vi "NI-Switch Main Page.vi"(8 "error in (no error)":errorcluster, 11 "Node Ptr":T1 format="%.0x") -> (0 "error out":errorcluster)   [LabVIEW 2010, in "NI-Switch Relay Custom Device.lvlib"]
uses:
  NI-Switch Relay Custom Device.lvlib
  <vilib>/NI Veristand/Custom Device API/Custom Device Item Ref.ctl
  NI-Switch Global.vi
  <vilib>/NI Veristand/Custom Device API/Get Item Property (String).vi
  <vilib>/NI Veristand/Custom Device API/Set Item Property (String).vi
  <vilib>/NI Veristand/Custom Device API/Custom Device API.lvlib
panel:
  out "Topology Name":string
  in  "Header 3":cluster{"Section Name":string}={"Section Name"="Custom Device Item Settings"}
  in  "Physical Address":string
  in  "Decimation":i32
  in  "Header 2":cluster{"Section Name":string}={"Section Name"="Custom Device Item Settings"}
  in  "Header":cluster{"Section Name":string}={"Section Name"="Custom Device Item Settings"}
  in  "Description":string
  in  "Name":string
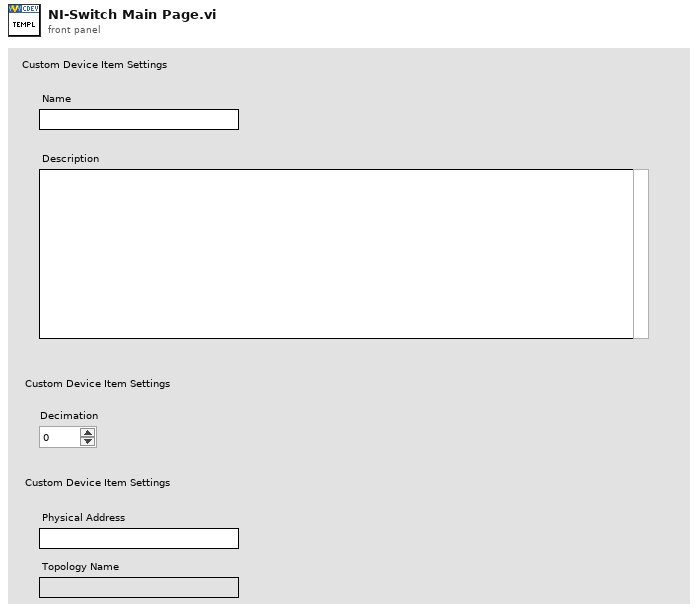
[diagram p1: front panel]
types:
  T1 = typedef "Custom Device API.lvlib/Custom Device Item Ref.ctl" = u64
  T2 = typedef "Custom Device API.lvlib/Custom Device Item Info.ctl" = cluster{"Name":string, "Is Channel":bool, "GUID":string}
  T3 = typedef "Custom Device API.lvlib/Custom Device Commands.ctl" = enum16{"Default", "Item renamed", "Shutdown", "Dynamic button pressed"}
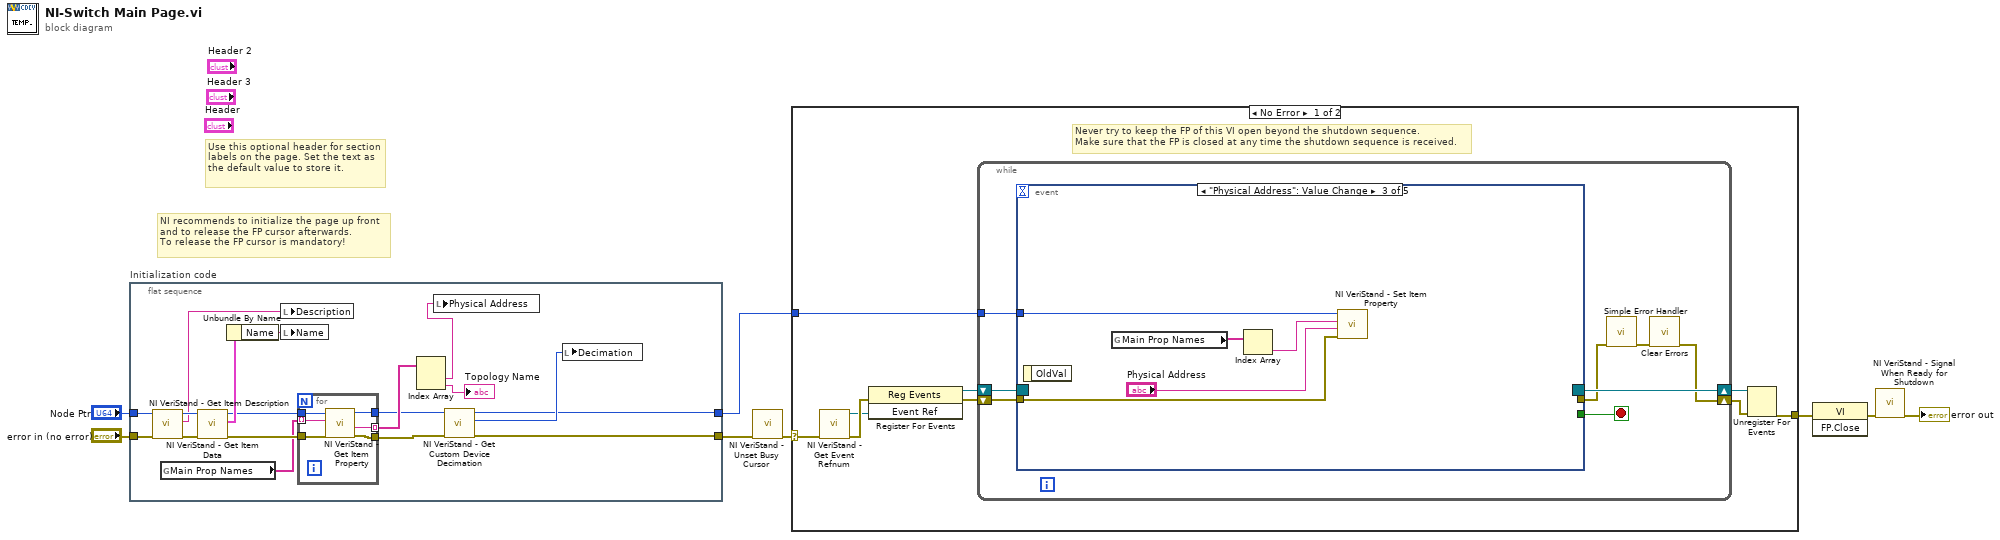
[diagram p0: block diagram]
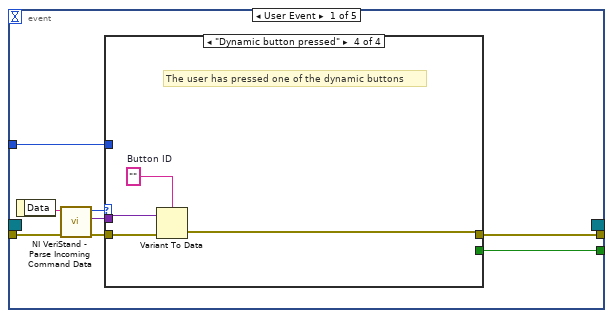
[diagram p2: hidden frame]
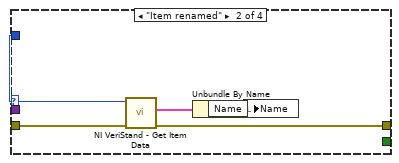
[diagram p4: hidden frame]
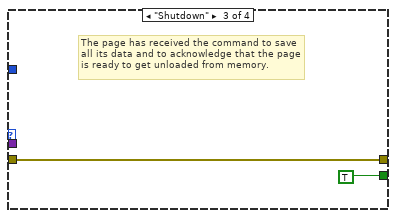
[diagram p5: hidden frame]
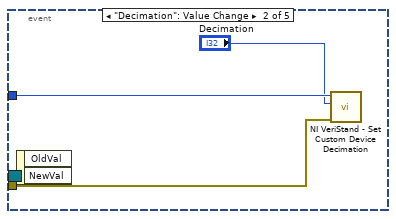
[diagram p6: hidden frame]
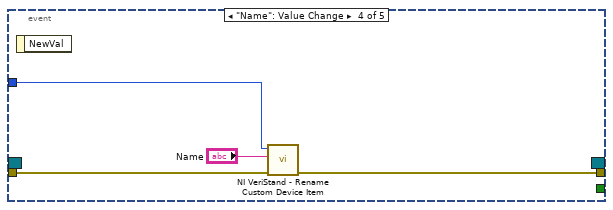
[diagram p7: hidden frame]
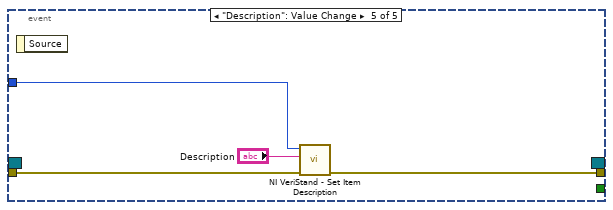
[diagram p8: hidden frame]
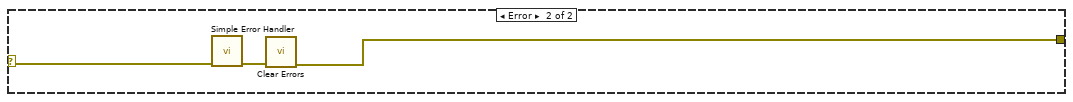
[diagram p9: hidden frame]
diagram:
  # "Use this optional header for section labels on the page. Set the text as the default value to store it."
  # "NI recommends to initialize the page up front\nand to release the FP cursor afterwards.\nTo release the FP cursor is mandatory!"
  n1 = flat-sequence "Initialization code" {
    tunnel: "error in (no error)" -> [w25]
    tunnel: "Node Ptr" -> [w24]
    tunnel: [w9] -> w4
    tunnel: [w10] -> w1
    frame #0 {
      n2 = call <vilib>:"NI VeriStand - Get Item Description.vi"("error in (no error)"=w25, "Item Ref in"=w24) -> ("error out"=w22:errorcluster, "Description"=w23:string, "Item Ref out"=w26:T1)  [unwired: 7 out]
      n3 = global read "NI-Switch Global.vi" "Main Prop Names"() -> (w17:string[])
      n4 = call <vilib>:"NI VeriStand - Get Item Data.vi"("error in (no error)"=w22, "Item Ref in"=w26) -> ("error out"=w18:errorcluster, "Item Info"=w21:T2, "Item Ref out"=w19:T1)  [unwired: 7 out]
      n5 = Unbundle By Name(w21) -> ("Name"=w20:string)
      n6 = local write "Description"(w23) -> ()
      n7 = local write "Name"(w20) -> ()
      n8 = for {
        tunnel: w19 -> [w32]
        tunnel: w18 -> [w31]
        tunnel: w17 -> [w30] mode=indexing
        tunnel: [w29] -> w16 mode=indexing
        tunnel: [w28] -> w13
        tunnel: [w27] -> w12
        n9 = call-poly <vilib>:"NI VeriStand - Get Item Property.vi"("error in (no error)"=w31, "Property Name"=w30, "Item Ref in"=w32) -> ("error out"=w27:errorcluster, "Value"=w29:string, "Item Ref out"=w28:T1)  [unwired: 5 in, 1 out]
      }
      n10 = Index Array(array=w16) -> (element #1=w14:string, element #2=→"Topology Name":string)  [unwired: 2 in]
      n11 = local write "Physical Address"(w14) -> ()
      n12 = call <vilib>:"NI VeriStand - Get Custom Device Decimation.vi"("error in (no error)"=w12, "Device Ref in"=w13) -> ("error out"=w9:errorcluster, "Decimation"=w11:i32, "Device Ref out"=w10:T1)  [unwired: 7 in]
      n13 = local write "Decimation"(w11) -> ()
    }
  }
  n14 = call <vilib>:"NI VeriStand - Unset Busy Cursor.vi"("error in (no error)"=w4) -> ("error out"=w3:errorcluster)  [unwired: 10 out]
  n15 = case shown="No Error" w3 {
    selector: w3 -> [w33 w88]
    tunnel: [w38 w86] -> w8
    tunnel: w1 -> [w34 _]
    frame No Error {
      # "Never try to keep the FP of this VI open beyond the shutdown sequence.\nMake sure that the FP is closed at any time the shutdown sequence is received."
      n16 = call <vilib>:"NI VeriStand - Get Event Refnum.vi"("error in (no error)"=w33) -> ("error out"=w41:errorcluster, "Event Ref"=w37:refnum<user-event>)  [unwired: 9 out]
      n17 = register-events(error in=w41, w37) -> (reference out=w35:refnum<event-registration>, error out=w36:errorcluster)  [unwired: 1 in]
      n18 = while {
        tunnel: w34 -> [w45]
        shift-right: [w42] -> w39
        shift-left: w36 -> [w48]
        shift-right: [w49] -> w40
        shift-left: w35 -> [w47]
        stop <- w46 stop-if-true
        n19 = event shown="[2] \"Physical Address\": Value Change" {
          selector: w47 -> [_ _ _ _ _]
          dyn-events: [_ _ _ _ _] -> w49
          timeout: _ -> [_ _ _ _ _]
          tunnel: w48 -> [w57 w70 w73 w81 w84]
          tunnel: [w53 _ _ _ _] -> w46
          tunnel: [w52 _ _ w80 w83] -> w44
          tunnel: w45 -> [w51 w72 w76 w79 w85]
          event User Event {
            n20 = event-data() -> ("Data"=w56:string)  [unwired: 1 out]
            n21 = call <vilib>:"NI VeriStand - Parse Incoming Command Data.vi"("error in (no error)"=w57, "Data"=w56) -> ("error out"=w55:errorcluster, "Data"=w50:variant, "Action"=w54:T3)  [unwired: 7 out]
            n22 = case shown="\"Dynamic button pressed\"" w54 {
              tunnel: w55 -> [w58 w63 w64 w69]
              tunnel: [_ _ TRUE _] -> w53
              tunnel: [w58 w60 w64 w66] -> w52
              tunnel: w51 -> [_ w62 _ _]
              tunnel: w50 -> [_ _ _ w68]
              frame "Default", Default {
              }
              frame "Item renamed" {
                n23 = call <vilib>:"NI VeriStand - Get Item Data.vi"("error in (no error)"=w63, "Item Ref in"=w62) -> ("error out"=w60:errorcluster, "Item Info"=w61:T2)  [unwired: 8 out]
                n24 = Unbundle By Name(w61) -> ("Name"=w59:string)
                n25 = local write "Name"(w59) -> ()
              }
              frame "Shutdown" {
                # "The page has received the command to save all its data and to acknowledge that the page is ready to get unloaded from memory."
              }
              frame "Dynamic button pressed" {
                w67 = ""  # Button ID
                # "The user has pressed one of the dynamic buttons"
                n26 = Variant To Data(error in=w69, Variant=w68, type=w67) -> (error out=w66:errorcluster)  [unwired: 1 out]
              }
            }
          }
          event "Decimation": Value Change {
            n27 = event-data() -> ()  [unwired: 3 out]
            n28 = call <vilib>:"NI VeriStand - Set Custom Device Decimation.vi"("error in (no error)"=w70, "Decimation"="Decimation", "Device Ref in"=w72) -> ()  [unwired: 7 in, 2 out]
          }
          event "Physical Address": Value Change {
            n29 = event-data() -> ()  [unwired: 2 out]
            n30 = global read "NI-Switch Global.vi" "Main Prop Names"() -> (w77:string[])
            n31 = Index Array(array=w77) -> (element=w74:string)  [unwired: 1 in]
            n32 = call-poly <vilib>:"NI VeriStand - Set Item Property.vi"("error in (no error)"=w73, "Value"="Physical Address", "Property Name"=w74, "Item Ref in"=w76) -> ()  [unwired: 5 in, 3 out]
          }
          event "Name": Value Change {
            n33 = event-data() -> ()  [unwired: 2 out]
            n34 = call <vilib>:"NI VeriStand - Rename Custom Device Item.vi"("error in (no error)"=w81, "New Name"="Name", "Item Ref in"=w79) -> ("error out"=w80:errorcluster)  [unwired: 8 out]
          }
          event "Description": Value Change {
            n35 = event-data() -> ()  [unwired: 2 out]
            n36 = call <vilib>:"NI VeriStand - Set Item Description.vi"("error in (no error)"=w84, "Description"="Description", "Item Ref in"=w85) -> ("error out"=w83:errorcluster)  [unwired: 8 out]
          }
        }
        n37 = call <vilib>:"Simple Error Handler.vi"("error in (no error)"=w44) -> ("error out"=w43:errorcluster)  [unwired: 1 in, 7 out]
        n38 = call <vilib>:"Clear Errors.vi"("error in (no error)"=w43) -> ("error out"=w42:errorcluster)  [unwired: 6 out]
      }
      n39 = Unregister For Events(event registration refnum=w40, error in=w39) -> (error out=w38:errorcluster)
    }
    frame Error {
      n40 = call <vilib>:"Simple Error Handler.vi"("error in (no error)"=w88) -> ("error out"=w87:errorcluster)  [unwired: 1 in, 7 out]
      n41 = call <vilib>:"Clear Errors.vi"("error in (no error)"=w87) -> ("error out"=w86:errorcluster)  [unwired: 6 out]
    }
  }
  n42 = invoke class="VI" method="FP.Close"(error in=w8) -> (error out=w7:errorcluster)  [unwired: 2 in, 2 out]
  n43 = call <vilib>:"NI VeriStand - Signal When Ready for Shutdown.vi"("error in (no error)"=w7) -> ("error out"=→"error out":errorcluster)  [unwired: 10 out]
